vi "Defeated Message.vi"(11 "MyTeam in":refnum<class "MyTeam.lvclass">) -> (2 "Defeated Message":string)   [LabVIEW 2020, in "Rain.lvlib" / "MyTeam.lvclass"]
uses:
  MyTeam.lvclass
  MyTeam.lvclass/MyTeam.ctl
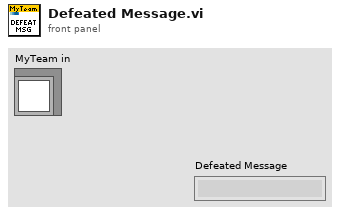
[diagram p1: front panel]
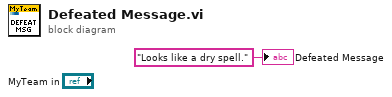
[diagram p0: block diagram]
diagram:
  "Defeated Message" <- "Looks like a dry spell." ("Defeated Message")
